vi "Go To Initial State.vi"(8 "error in (no error)":errorcluster, 11 "ConnectCommand in":refnum<class "Connect Command.lvclass">=refnum) -> (0 "error out":errorcluster, 3 "State Actor.lvclass":refnum<class "State Actor.lvclass">)   [LabVIEW 2013, in "Receiver.lvlib" / "Receive Commands Using State Actors.lvlib" / "Connect Command.lvlib" / "Connect Command.lvclass"]
uses:
  Connect Command/Connect Command.lvclass
  <vilib>/ni/Actors/State Actor/State Actor/State Actor.lvclass
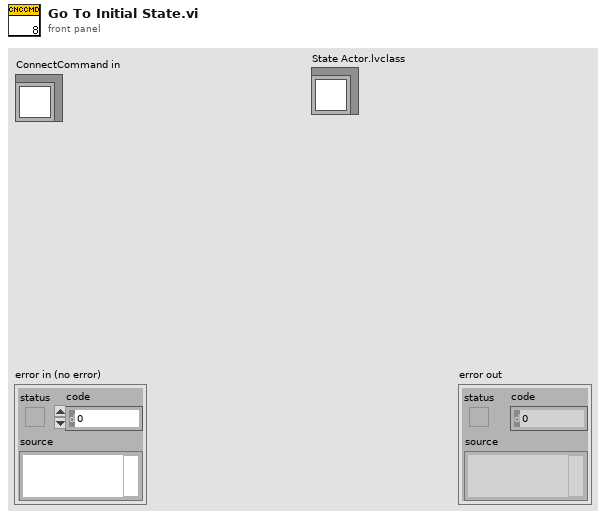
[diagram p1: front panel]
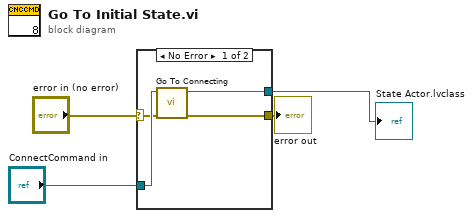
[diagram p0: block diagram]
diagram:
  n1 = case shown="No Error" "error in (no error)" {
    selector: "error in (no error)" -> [w7 w10]
    tunnel: [w6 w10] -> w3
    tunnel: "ConnectCommand in" -> [w8 w9]
    tunnel: [w5 w9] -> w1
    frame No Error {
      n2 = call-dynamic "Go To Connecting.vi"("error in (no error)"=w7, "ConnectCommand in"=w8) -> ("error out"=w6:errorcluster, "State Actor.lvclass"=w5:refnum<class "State Actor.lvclass">)  [unwired: 8 in]
    }
    frame Error {
    }
  }
  "error out" <- w3
  "State Actor.lvclass" <- w1
